vi "Create MB Address Block.vi"(8 "Number of Registers in Block":u16, 9 "Start Address":u16, 10 "Modbus Address Type":T1="0", 11 "Base Address URL":string) -> (1 "Starting Address (SGL)":i32, 3 "Modbus URL":string)   [LabVIEW 2012, in "Configuration Grandmaster.lvlib" / "TimingGrp.lvclass"]
doc: "This VI creates a modbus block URL for the NI Modbus IO Server using a Base Address URL, a Modbus Address Type, a Start Address, and the Number of Registers in Block. \n\nThe Start Address and Number of Registers in Block inputs must both be greater than zero or else the VI will return an empty string.\n\nThis VI uses the address definition defined by the NI Modbus IO Server defined here:\nhttp://zone.ni.com/reference/en-XX/help/371618F-01/lvmve/dsc_modbus_using/"
uses:
  TimingGrp.lvclass
  Custom Ctrls/Modbus Address Header.ctl
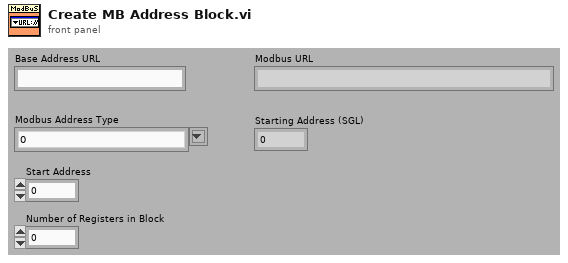
[diagram p1: front panel]
types:
  T1 = typedef "Modbus Address Header.ctl" = string
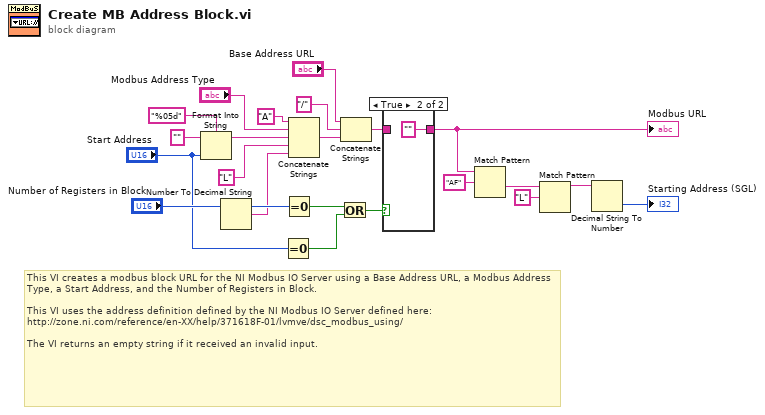
[diagram p0: block diagram]
diagram:
  # "This VI creates a modbus block URL for the NI Modbus IO Server using a Base Address URL, a Modbus Address Type, a Start Address, and the Number of Registers in Block.  \n\nThis VI uses the address definition defined by the NI Modbus IO Server defined here:\nhttp://zone.ni.com/reference/en-XX/help/371618F-01/lvmve/dsc_modbus_using/ \n\nThe VI returns an empty string if it received an invalid input."
  n1 = Format Into String(format string="%05d", initial string="", "Start Address") -> (resulting string=w11:string)  [unwired: 1 in, 1 out]
  n2 = Number To Decimal String(number="Number of Registers in Block") -> (decimal integer string=w17:string)  [unwired: 1 in]
  n3 = Equal To 0?(x="Start Address") -> (x = 0?=w8:bool)
  n4 = Equal To 0?(x="Number of Registers in Block") -> (x = 0?=w9:bool)
  n5 = Concatenate Strings("A" ("string"), "Modbus Address Type", w11, "L" ("string"), w17) -> (w14:string)
  n6 = Or(x=w9, y=w8) -> (x .or. y?=w7:bool)
  n7 = Concatenate Strings("Base Address URL", "/" ("string"), w14) -> (w15:string)
  n8 = case shown="True" w7 {
    tunnel: w15 -> [w23 _]
    tunnel: [w23 ""] -> w2
    frame False {
    }
    frame True {
    }
  }
  "Modbus URL" <- w2
  n9 = Match Pattern(string=w2, regular expression="AF") -> (after substring=w5:string)  [unwired: 1 in, 3 out]
  n10 = Match Pattern(string=w5, regular expression="L") -> (before substring=w3:string)  [unwired: 1 in, 3 out]
  n11 = Decimal String To Number(string=w3) -> (number=→"Starting Address (SGL)":i32)  [unwired: 2 in, 1 out]
